vi "S2C_OM8257_Proc_Status.vi"(8 "Error In":errorcluster) -> (0 "Error Out":errorcluster, 3 "Response":string)   [LabVIEW 2015]
uses:
  S2C_OM8257_Proc_Globals.vi
  <instrlib>/Associated Research 82XX/Associated Research 82XX.lvlib
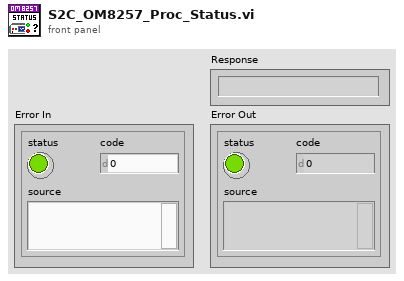
[diagram p1: front panel]
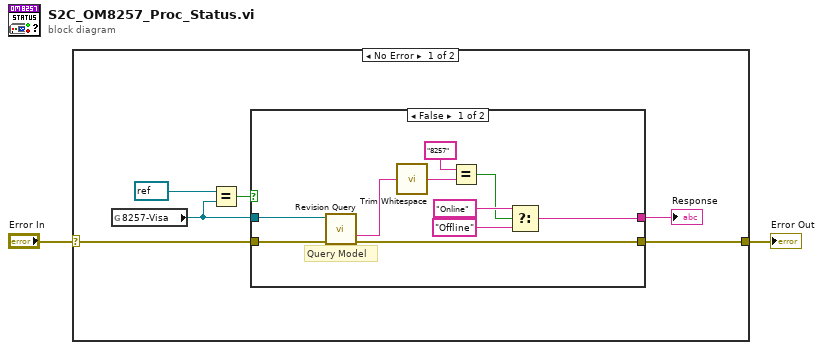
[diagram p0: block diagram]
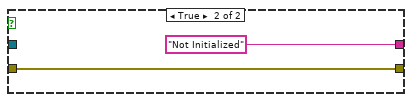
[diagram p2: hidden frame]
diagram:
  n1 = case shown="No Error" "Error In" {
    selector: "Error In" -> [w8 w21]
    tunnel: [w7 w21] -> w1
    frame No Error {
      n2 = global read "S2C_OM8257_Proc_Globals.vi" "8257-Visa"() -> (w3:refnum<visa-resource-name>)
      n3 = Equal?(x=refnum<visa-resource-name> refnum ("SerialRef"), y=w3) -> (x = y?=w4:bool)
      n4 = case shown="False" w4 {
        tunnel: w8 -> [w15 w20]
        tunnel: w3 -> [w14 _]
        tunnel: [w10 w20] -> w7
        tunnel: [w16 "Not Initialized" ("f")] -> w6
        frame False {
          # "Query Model"
          n5 = call <instrlib>:"Revision Query.vi"("VISA resource name"=w14, "error in (no error)"=w15) -> ("Instrument Model"=w13:string, "error out"=w10:errorcluster)  [unwired: 9 in, 3 out]
          n6 = call <vilib>:"Trim Whitespace.vi"("string"=w13) -> ("trimmed string"=w11:string)  [unwired: 1 in]
          n7 = Equal?(x="8257", y=w11) -> (x = y?=w9:bool)
          n8 = Select(t="Online", s=w9, f="Offline") -> (s? t:f=w16:string)
        }
        frame True {
        }
      }
      "Response" <- w6
    }
    frame Error {
    }
  }
  "Error Out" <- w1
